vi "TCP_Controller.vi"() -> ()   [LabVIEW 2021]
panel:
  out "error out":errorcluster
  in  "error in (no error)":errorcluster
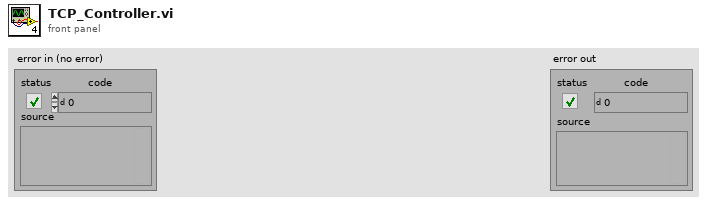
[diagram p1: front panel]
types:
  T1 = enum32{"Invalid", "Standard", "Closed", "Hidden", "Minimized", "Maximized"}
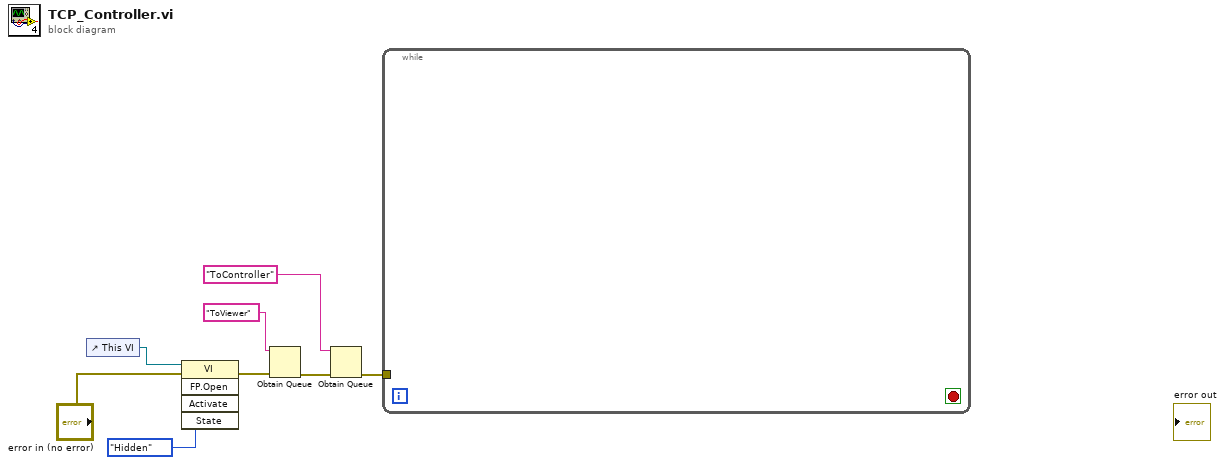
[diagram p0: block diagram]
diagram:
  n1 = control-ref of="This VI"() -> (w8:refnum<vi>)
  n2 = invoke class="VI" method="FP.Open"(reference=w8, error in="error in (no error)", "State"=T1."Hidden") -> (error out=w5:errorcluster)  [unwired: 2 in, 4 out]
  n3 = Obtain Queue(name (unnamed)="ToViewer", error in (no error)=w5) -> (error out=w4:errorcluster)  [unwired: 3 in, 2 out]
  n4 = Obtain Queue(name (unnamed)="ToController", error in (no error)=w4) -> (error out=w2:errorcluster)  [unwired: 3 in, 2 out]
  n5 = while {
    tunnel: w2 -> [_]
    stop <- _ stop-if-true
  }
